vi "SetEnableBySignalName.vi"(9 "State":bool, 10 "Signal Name":string, 11 "Trigger Data Input":T3) -> (3 "Trigger Data Output":T3)   [LabVIEW 2016]
uses:
  Ctrl_Signal.ctl
  Ctrl_Signal_Map.ctl
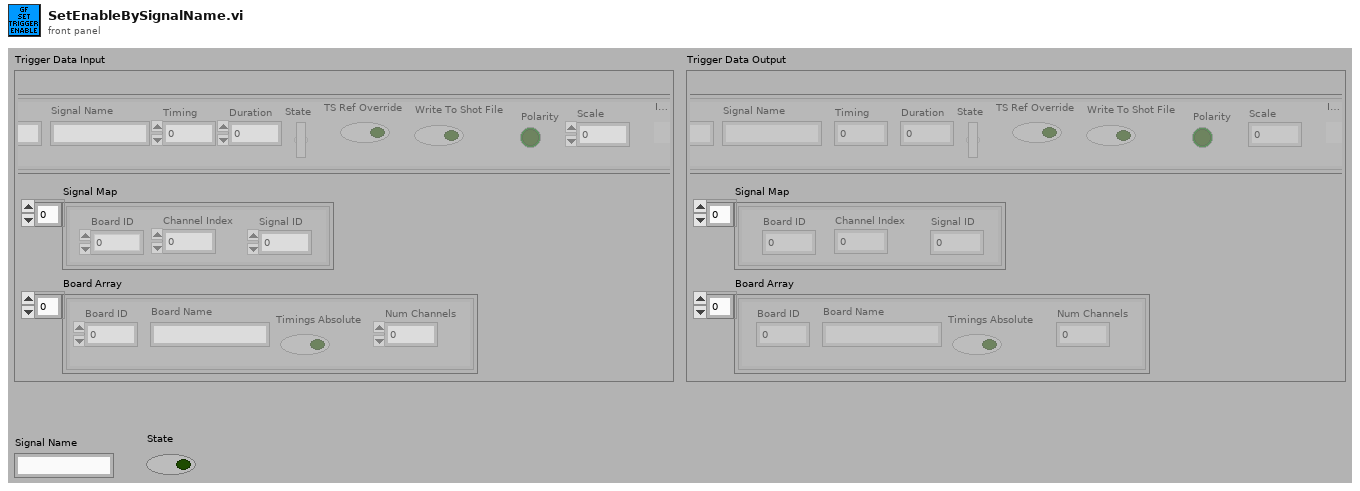
[diagram p1: front panel]
types:
  T1 = typedef "Ctrl_Signal.ctl" = cluster{"Signal Name":string, "Timing":dbl, "Duration":dbl, "State":bool, "TS Ref Override":bool, "Write To Shot File":bool, "Polarity":bool, "Signal ID":dbl, "Scale":dbl, "IsDelay":bool}
  T2 = typedef "Ctrl_Signal_Map.ctl" = cluster{"Channel Index":dbl, "Board ID":dbl, "Signal ID":dbl}
  T3 = cluster{"Signal Array":T1[], "Signal Map":T2[], "Board Array":cluster{"Board ID":dbl, "Board Name":string, "Timings Absolute":bool, "Num Channels":dbl}[]}
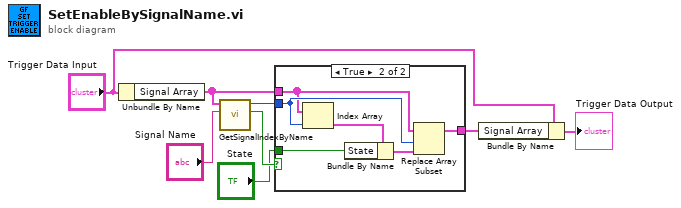
[diagram p0: block diagram]
diagram:
  n1 = Unbundle By Name("Trigger Data Input") -> ("Signal Array"=w1:T1[])
  n2 = call "GetSignalIndexByName.vi"("Signal Name"="Signal Name", "Signal Array In"=w1) -> ("Signal Found"=w7:bool, "Index Out"=w6:u32)  [unwired: 8 in]
  n3 = case shown="True" w7 {
    tunnel: w1 -> [w9 w11]
    tunnel: w6 -> [_ w13]
    tunnel: "State" -> [_ w14]
    tunnel: [w9 w10] -> w2
    frame False {
    }
    frame True {
      n4 = Index Array(array=w11, index=w13) -> (element=w15:T1)
      n5 = Bundle By Name(cluster=w15, "State"=w14) -> (w12:T1)
      n6 = Replace Array Subset(array=w11, new element=w12, index=w13) -> (w10:T1[])
    }
  }
  n7 = Bundle By Name(cluster="Trigger Data Input", "Signal Array"=w2) -> (→"Trigger Data Output":T3)
